vi "GenerateUniqueFilename.vi"(5 "Index digits":i32=3, 7 "format string":string, 8 "Error In":errorcluster, 9 "File name suffixes":string[](array[string]), 11 "Folder Path Control":path) -> (0 "Error Out":errorcluster, 1 "Index out":i32=-1, 2 "Try count":i32, 3 "Paths":path[](array[path]))   [LabVIEW 2024]
panel:
  out "Any file exists?":bool
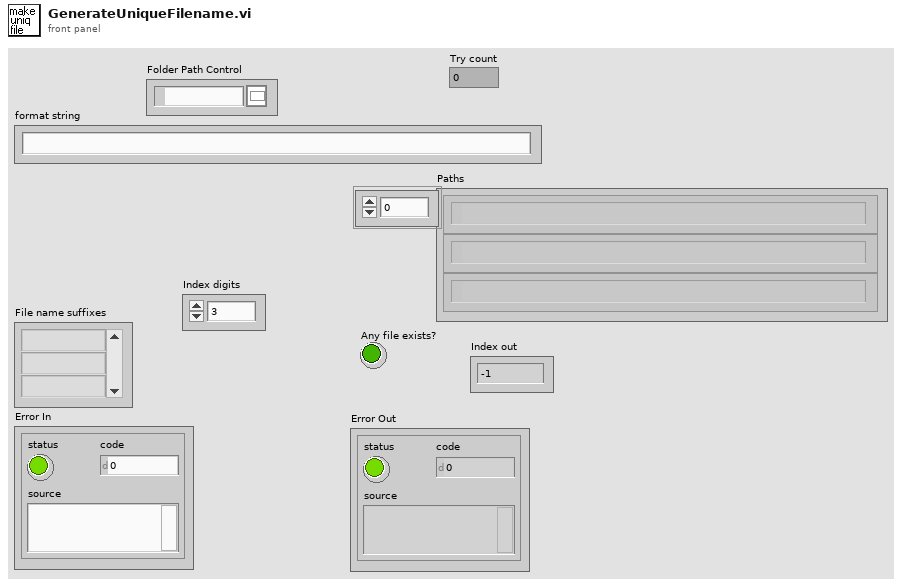
[diagram p1: front panel]
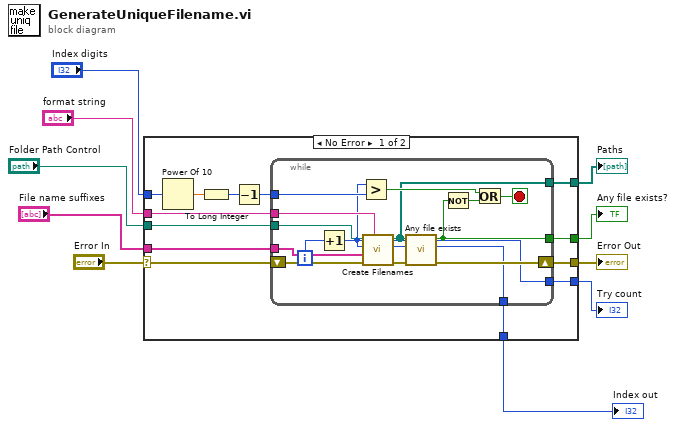
[diagram p0: block diagram]
diagram:
  n1 = case shown="No Error" "Error In" {
    selector: "Error In" -> [w22 w39]
    tunnel: [w23 w39] -> w9
    tunnel: "Index digits" -> [w21 _]
    tunnel: "Folder Path Control" -> [w17 _]
    tunnel: [w16 _] -> w6
    tunnel: [w15 _] -> w5
    tunnel: "format string" -> [w14 _]
    tunnel: "File name suffixes" -> [w13 _]
    tunnel: [w12 _] -> w2
    tunnel: [w11 _] -> w1
    frame No Error {
      n2 = Power Of 10(x=w21) -> (10^x=w20:dbl)
      n3 = To Long Integer(number=w20) -> (32bit integer=w19:i32)
      n4 = Decrement(x=w19) -> (x-1=w18:i32)
      n5 = while {
        tunnel: [w29] -> w15
        shift-right: [w37] -> w23
        shift-left: w22 -> [w27]
        tunnel: w18 -> [w36]
        tunnel: w17 -> [w31]
        tunnel: [w33] -> w16
        tunnel: w14 -> [w32]
        tunnel: w13 -> [w28]
        tunnel: [w25] -> w12
        tunnel: [w24] -> w11
        i -> [w33]
        stop <- w38 stop-if-true
        n6 = Increment(x=w33) -> (x+1=w30:i32)
        n7 = Greater?(x=w30, y=w36) -> (0:w34:bool)
        n8 = call "Create Filenames.vi"("Format string"=w32, "Error In"=w27, "File name suffixes"=w28, "Index"=w30, "Folder Path Control"=w31) -> ("Error Out"=w26:errorcluster, "Index out"=w24:i32, "Paths"=w29:path[])  [unwired: 4 in]
        n9 = call "Any file exists.vi"("Error In"=w26, "Files"=w29) -> ("Error Out"=w37:errorcluster, "Any file exists?"=w25:bool)  [unwired: 8 in]
        n10 = Not(x=w25) -> (.not. x?=w35:bool)
        n11 = Or(x=w34, y=w35) -> (x .or. y?=w38:bool)
      }
    }
    frame Error {
    }
  }
  "Error Out" <- w9
  "Try count" <- w6
  "Paths" <- w5
  "Any file exists?" <- w2
  "Index out" <- w1
